vi "Global 1.vi"() -> ()   [LabVIEW 2020]
panel:
  in  "Median Filter Rank":i32=5
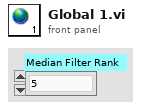
[diagram p1: front panel]
diagram:
